vi "Model_New.vi"(8 "error in (no error)":errorcluster caption="错误输入（无错误）", 11 "User Management Model 输入":refnum<class "User Management Model.lvclass">) -> (0 "error out":errorcluster caption="错误输出", 3 "User Management Model 输出":refnum<class "User Management Model.lvclass">)   [LabVIEW 2019, in "User Management Model.lvclass"]
uses:
  User Management Model.lvclass
  protect/ObjectAttributes.ctl
  User Management Model.lvclass/User Management Model.ctl
panel:
  in  "Attributes":T1
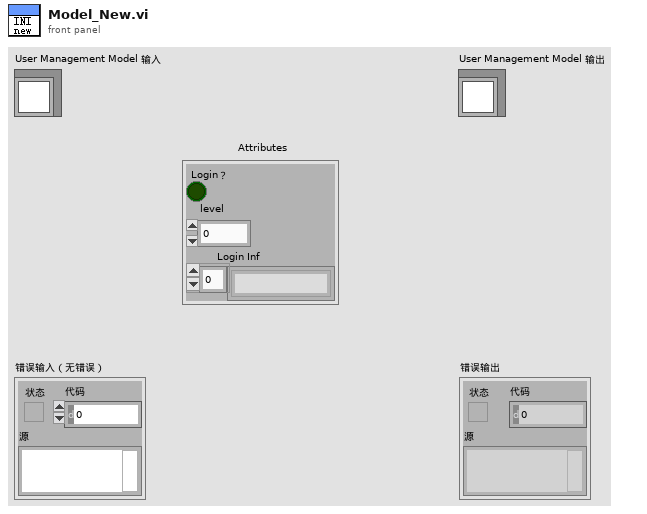
[diagram p1: front panel]
types:
  T1 = typedef "User Management Model.lvclass/ObjectAttributes.ctl" = cluster{"Login？":bool, "level":i32, "Login Inf":string[]}
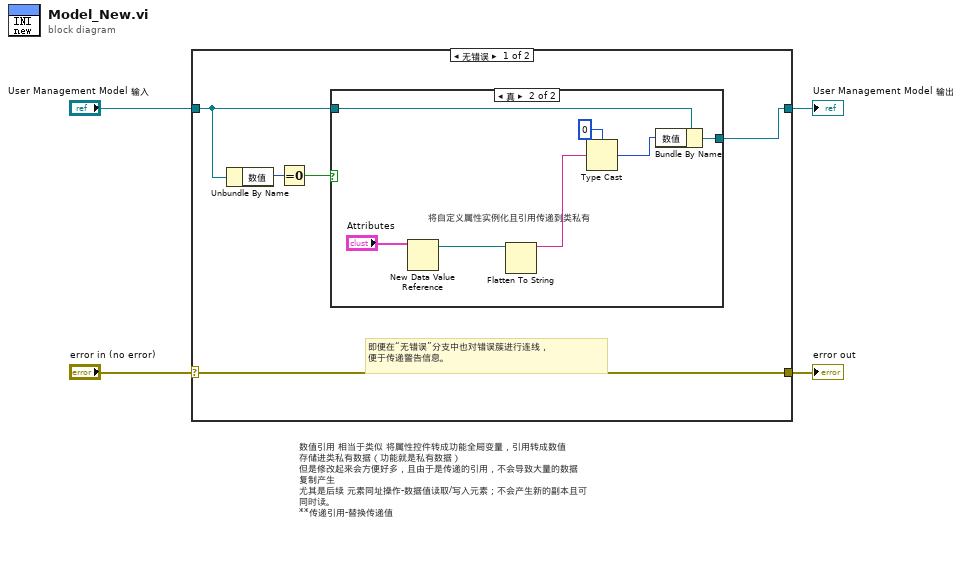
[diagram p0: block diagram]
diagram:
  # "数值引用 相当于类似 将属性控件转成功能全局变量，引用转成数值\n存储进类私有数据（功能就是私有数据）\n但是修改起来会方便好多，且由于是传递的引用，不会导致大量的数据\n复制产生\n尤其是后续 元素同址操作-数据值读取/写入元素；不会产生新的副本且可\n同时读。\n**传递引用-替换传递值"
  n1 = case shown="无错误" "error in (no error)" {
    selector: "error in (no error)" -> [w9 w19]
    tunnel: [w9 w19] -> w3
    tunnel: [w8 w18] -> w1
    tunnel: "User Management Model 输入" -> [w7 w18]
    frame No Error {
      # "即便在“无错误”分支中也对错误簇进行连线，\n便于传递警告信息。"
      n2 = Unbundle By Name(w7) -> ("数值"=w6:u32)
      n3 = Equal To 0?(x=w6) -> (x = 0?=w5:bool)
      n4 = case shown="真" w5 {
        tunnel: [w10 w17] -> w8
        tunnel: w7 -> [w10 w11]
        frame False {
          # "存在引用值，不再生成引用值"
        }
        frame True {
          # "将自定义属性实例化且引用传递到类私有"
          n5 = New Data Value Reference(data value="Attributes") -> (data value reference=w15:refnum<data-value>)  [unwired: 1 in, 1 out]
          n6 = Flatten To String(anything=w15) -> (data string=w14:string)  [unwired: 3 in, 2 out]
          n7 = Type Cast(type=u32 0 ("数值"), x=w14) -> (*(type *) &x=w12:u32)
          n8 = Bundle By Name(cluster=w11, "数值"=w12) -> (w17:refnum<class "User Management Model.lvclass">)
        }
      }
    }
    frame Error {
    }
  }
  "error out" <- w3
  "User Management Model 输出" <- w1
